vi "Create Caster Wheel.vi"(4 "caster motor communication":refnum<class "NI_Robotics_Motor Communication.lvclass">, 6 "motor communication":refnum<class "NI_Robotics_Motor Communication.lvclass">, 7 "caster parameters":T1={"forward offset"=0.0, "caster gear ratio"=1.0}, 8 "error in (no error)":errorcluster, 10 "wheel name":string, 11 "wheel parameters":T2={"wheel radius"=1.0, "gear ratio"=1.0, "forward rotation direction"=0} {"forward rotation direction" items=["Clockwise", "Counterclockwise"]}) -> (0 "error out":errorcluster, 3 "caster wheel out":refnum<class "NI_Robotics_Caster Wheel.lvclass">)   [LabVIEW 2017, in "NI_Robotics_Caster Wheel.lvclass"]
doc: "Creates a wheel of the type you specify that you can add to a steering frame. You must manually select the polymorphic instance to use."
uses:
  <vilib>/robotics/Steering/Caster Wheel/NI_Robotics_Caster Wheel.lvclass
  c:/Program Files (x86)/National Instruments/LabVIEW 2017/vi.lib/robotics/Steering/Wheel/NI_Robotics_Wheel.lvclass
  <vilib>/robotics/Steering/Wheel/Wheel Parameters.ctl
  <vilib>/robotics/Steering/Wheel/Rotation Direction.ctl
  <vilib>/robotics/Actuation/Motor Communication/NI_Robotics_Motor Communication.lvclass
  <vilib>/robotics/Steering/Caster Wheel/Caster Wheel Parameters.ctl
  <vilib>/robotics/Actuation/Motor Communication/NI_Robotics_Motor Communication.lvclass/NI_Robotics_Motor Communication.ctl
  <vilib>/robotics/Steering/Wheel/NI_Robotics_Wheel.lvclass/NI_Robotics_Wheel.ctl
  <vilib>/robotics/Steering/Caster Wheel/NI_Robotics_Caster Wheel.lvclass/NI_Robotics_Caster Wheel.ctl
  <vilib>/robotics/Actuation/Motor Communication/Get Initialized State.vi
  <vilib>/robotics/Actuation/Motor Communication Val/NI_Robotics_Motor Communication Val.lvclass
  c:/Program Files (x86)/National Instruments/LabVIEW 2017/vi.lib/robotics/Actuation/Motor Communication/NI_Robotics_Motor Communication.lvclass
  <vilib>/robotics/Actuation/Motor Communication Val/Initialize Motor Communication Val.vi
  <vilib>/robotics/Steering/Wheel/NI_Robotics_Wheel.lvclass
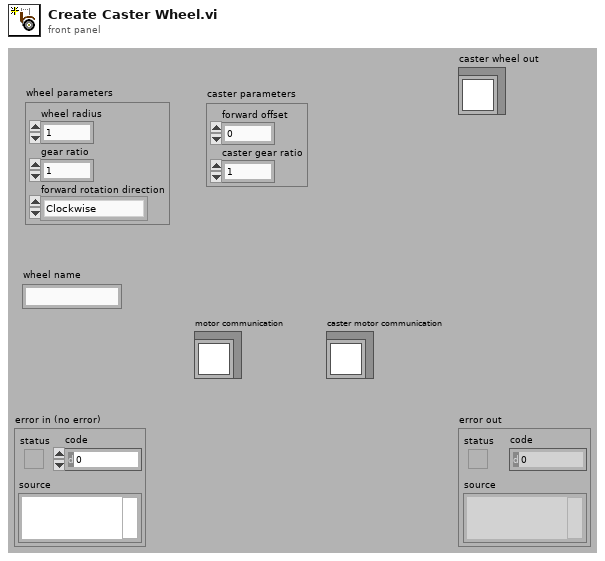
[diagram p1: front panel]
types:
  T1 = typedef "NI_Robotics_Caster Wheel.lvclass/Caster Wheel Parameters.ctl" = cluster{"forward offset":dbl, "caster gear ratio":dbl}
  T2 = typedef "NI_Robotics_Wheel.lvclass/Wheel Parameters.ctl" = cluster{"wheel radius":dbl, "gear ratio":dbl, "forward rotation direction":T3}
  T3 = typedef "NI_Robotics_Wheel.lvclass/Rotation Direction.ctl" = u16
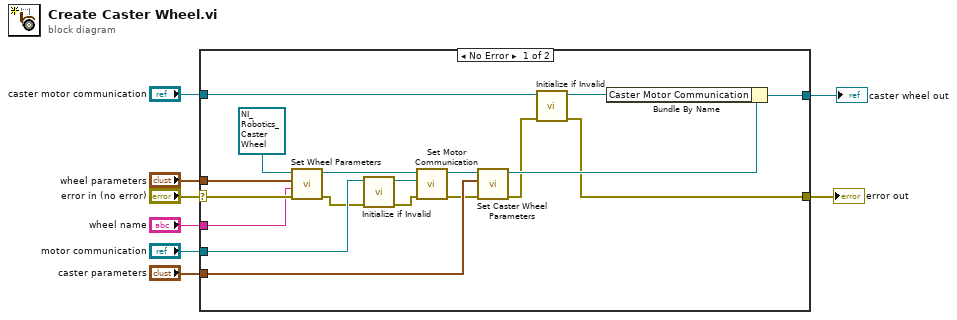
[diagram p0: block diagram]
diagram:
  n1 = case shown="No Error" "error in (no error)" {
    selector: "error in (no error)" -> [w25 w27]
    tunnel: [w9 w27] -> w7
    tunnel: "wheel parameters" -> [w24 _]
    tunnel: "motor communication" -> [w16 _]
    tunnel: "caster parameters" -> [w23 _]
    tunnel: "caster motor communication" -> [w12 _]
    tunnel: [w21 _] -> w2
    tunnel: "wheel name" -> [w20 _]
    frame No Error {
      n2 = call <vilib>:"Set Wheel Parameters.vi"("error in (no error)"=w25, "wheel name"=w20, "wheel parameters"=w24, "wheel in"=refnum<class "NI_Robotics_Caster Wheel.lvclass"> refnum ("CasterWheel in")) -> ("error out"=w13:errorcluster, "wheel out"=w19:refnum<class "NI_Robotics_Caster Wheel.lvclass">)  [unwired: 6 in]
      n3 = call <vilib>:"Initialize if Invalid.vi"("error in (no error)"=w13, "motor communication in"=w16) -> ("error out"=w14:errorcluster, "motor communication out"=w15:refnum<class "NI_Robotics_Motor Communication.lvclass">)  [unwired: 7 in, 1 out]
      n4 = call <vilib>:"Set Motor Communication.vi"("error in (no error)"=w14, "motor communication"=w15, "wheel in"=w19) -> ("error out"=w17:errorcluster, "wheel out"=w18:refnum<class "NI_Robotics_Caster Wheel.lvclass">)  [unwired: 7 in]
      n5 = call <vilib>:"Set Caster Wheel Parameters.vi"("error in (no error)"=w17, "caster parameters"=w23, "caster wheel in"=w18) -> ("error out"=w10:errorcluster, "caster wheel out"=w22:refnum<class "NI_Robotics_Caster Wheel.lvclass">)  [unwired: 7 in]
      n6 = call <vilib>:"Initialize if Invalid.vi"("error in (no error)"=w10, "motor communication in"=w12) -> ("error out"=w9:errorcluster, "motor communication out"=w11:refnum<class "NI_Robotics_Motor Communication.lvclass">)  [unwired: 7 in, 1 out]
      n7 = Bundle By Name(cluster=w22, "Caster Motor Communication"=w11) -> (w21:refnum<class "NI_Robotics_Caster Wheel.lvclass">)
    }
    frame Error {
    }
  }
  "error out" <- w7
  "caster wheel out" <- w2
